vi "set_plot_rjx.vi"(0 "enable_plot_jx":bool, 1 "set_scale":bool, 5 "enable_plot_jxp":bool, 7 "enable_plot_r":bool, 9 "enable_plot_rp":bool, 11 "enable_plot_z":bool, 12 "plot_rjx_ref":refnum<vi>, 14 "rx_scale_settings":enum32{"autoscale", "fancy_scale"}(ring)) -> ()   [LabVIEW 2025]
uses:
  281b8575-583e-44d6-aa3f-c5897071c9fa.vi
  b1141ece-3948-4364-a748-8af99b6ed624.vi
  889c7458-1fcf-4721-b08b-31ed2256c1a7.vi
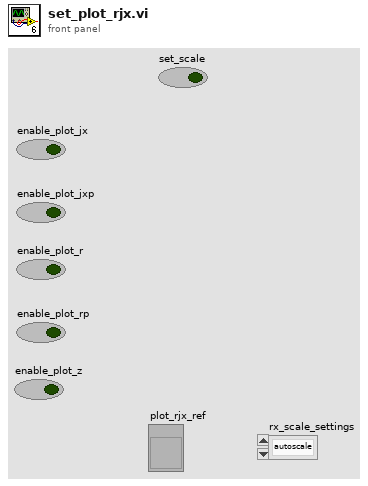
[diagram p1: front panel]
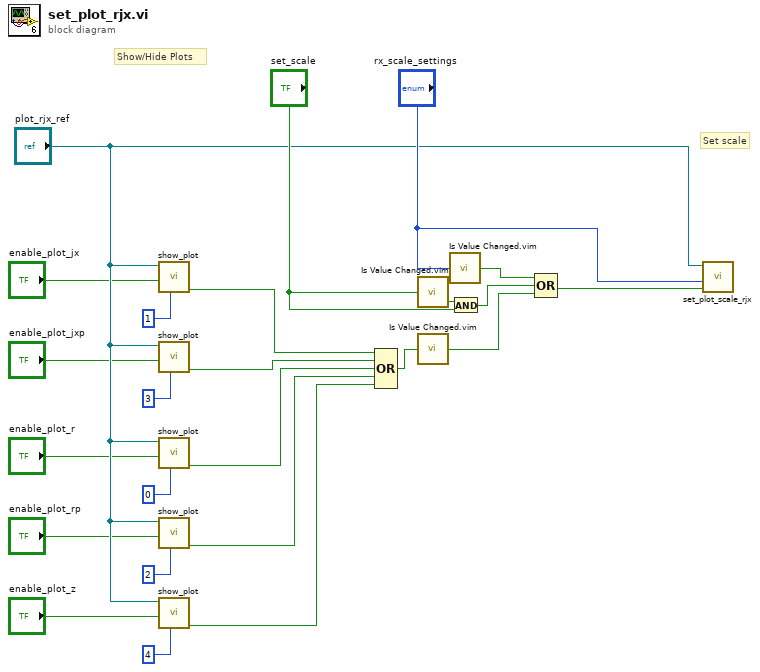
[diagram p0: block diagram]
diagram:
  # "Set scale"
  # "Show/Hide Plots"
  n1 = call "show_plot.vi"("plot_id"=1 ("y_scale_id"), "show_plot"="enable_plot_jx", "XYGraph Refnum"="plot_rjx_ref") -> ("done"=w5:bool)  [unwired: 8 in]
  n2 = call "show_plot.vi"("plot_id"=3 ("y_scale_id"), "show_plot"="enable_plot_jxp", "XYGraph Refnum"="plot_rjx_ref") -> ("done"=w4:bool)  [unwired: 8 in]
  n3 = call "show_plot.vi"("plot_id"=0 ("y_scale_id"), "show_plot"="enable_plot_r", "XYGraph Refnum"="plot_rjx_ref") -> ("done"=w3:bool)  [unwired: 8 in]
  n4 = call "show_plot.vi"("plot_id"=2 ("y_scale_id"), "show_plot"="enable_plot_rp", "XYGraph Refnum"="plot_rjx_ref") -> ("done"=w2:bool)  [unwired: 8 in]
  n5 = call "show_plot.vi"("plot_id"=4 ("y_scale_id"), "show_plot"="enable_plot_z", "XYGraph Refnum"="plot_rjx_ref") -> ("done"=w1:bool)  [unwired: 8 in]
  n6 = Compound Arithmetic op=OR(w5, w4, w3, w2, w1) -> (w11:bool)
  n7 = call "Is Value Changed.vim"("value"="set_scale") -> ("changed or first call?"=w20:bool)
  n8 = call "Is Value Changed.vim"("value"=w11) -> ("changed or first call?"=w21:bool)
  n9 = call "Is Value Changed.vim"("value"="rx_scale_settings") -> ("changed or first call?"=w19:bool)
  n10 = And(x=w20, y="set_scale") -> (x .and. y?=w18:bool)
  n11 = Compound Arithmetic op=OR(w19, w18, w21) -> (w23:bool)
  n12 = call "set_plot_scale_rjx.vi"("set_scale"=w23, "rx_scale_settings"="rx_scale_settings", "plot_rjx_ref"="plot_rjx_ref") -> ()  [unwired: 9 in]
